vi "DBL Array to Result 2.vi"(7 "Result name":string, 8 "Error In":errorcluster, 10 "Data":dbl[](array[numeric]), 11 "Channel Names":string[](array[string])) -> (0 "Error Out":errorcluster, 3 "Mag Lab Result out":refnum<class "Mag Lab Result.lvclass">)   [LabVIEW 2015]
uses:
  Mag Lab Result.lvclass
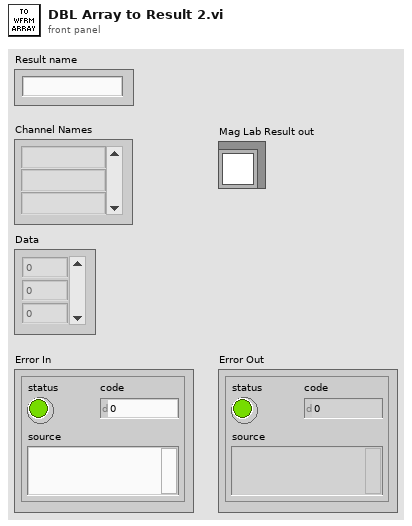
[diagram p1: front panel]
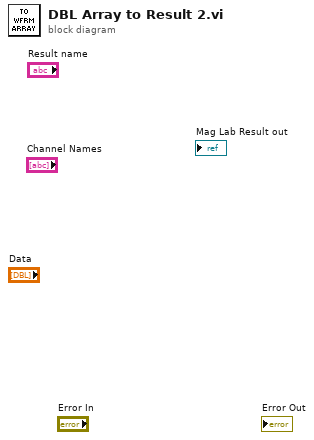
[diagram p0: block diagram]
diagram:
